vi "Strip HTML.vi"(8 "error in":errorcluster, 11 "HTML String":string) -> (0 "error out":errorcluster, 1 "HTML Stripped String":string, 3 "HTML String OUT":string, 4 "HTML Code Offsets":i32[](array[numeric]), 5 "HTML Codes":string[](array[string]))   [LabVIEW 2017]
doc: "This VI parses an HTML string and removes HTML <...> style tags. The HTML Tag Array contains clusters of the found tags and their corresponding indexes in the original HTML string.\n\nAlso replaces:\n o &nbsp; with \" \" ( a space)\n o &amp; with \"&\"\n\nTypical use of the HTML Tag Array is to locate sections of the HTML code to perform specific operations.\n\nRev 0.0.0 07/09/2009 Phillip Brooks\n Originated."
uses:
  <vilib>/regexp/Match Regular Expression.xnode
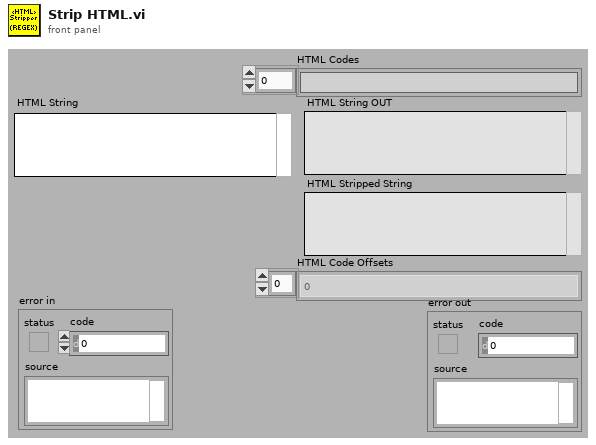
[diagram p1: front panel]
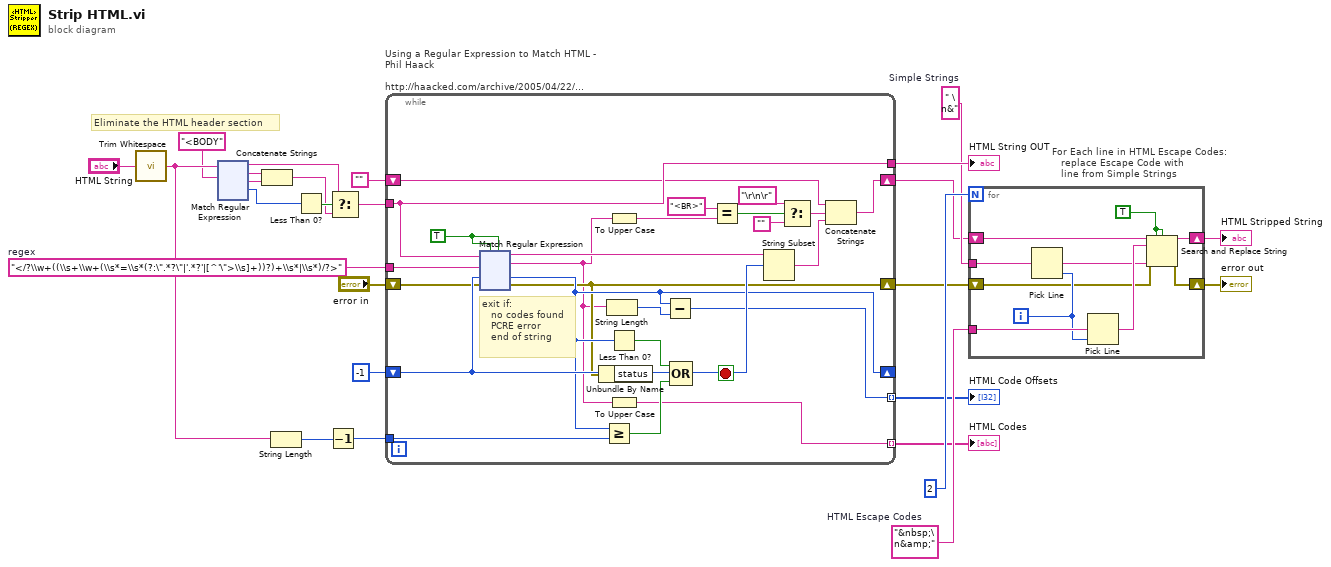
[diagram p0: block diagram]
diagram:
  w17 = " \n&"  # Simple Strings
  w19 = "&nbsp;\n&amp;"  # HTML Escape Codes
  w24 = "</?\\w+((\\s+\\w+(\\s*=\\s*(?:\".*?\"|'.*?'|[^'\">\\s]+))?)+\\s*|\\s*)/?>"  # regex
  # "Eliminate the HTML header section"
  n1 = call <vilib>:"Trim Whitespace.vi"("string"="HTML String") -> ("trimmed string"=w9:string)  [unwired: 1 in]
  n2 = xnode "Match Regular Expression"("input string"=w9, "regular expression"="<BODY") -> ("before match"=w3:string, "whole match"=w6:string, "after match"=w7:string, "offset past match"=w5:i32)  [unwired: 2 in, 3 out]
  n3 = Concatenate Strings(w6, w7) -> (w2:string)
  n4 = String Length(string=w9) -> (length=w22:i32)
  n5 = Less Than 0?(x=w5) -> (x < 0?=w4:bool)
  n6 = Decrement(x=w22) -> (x-1=w21:i32)
  n7 = Select(t=w3, s=w4, f=w2) -> (s? t:f=w1:string)
  n8 = while "Using a Regular Expression to Match HTML - Phil Haack\n\nhttp://haacked.com/archive/2005/04/22/Matching_HTML_With_Regex.aspx" {
    tunnel: w24 -> [w52]
    shift-right: [w44] -> _
    shift-left: -1 -> [w48]
    tunnel: w1 -> [w41]
    shift-right: [w49] -> w16
    shift-left: "" -> [w30]
    tunnel: w21 -> [w43]
    tunnel: [w41] -> w20
    tunnel: [w38] -> w14 mode=indexing
    tunnel: [w39] -> w13 mode=indexing
    shift-right: [w36] -> w11
    shift-left: "error in" -> [w37]
    stop <- w46 stop-if-true
    w40 = TRUE ("ignore case? (F)")
    # "exit if:\n   no codes found\n   PCRE error\n   end of string"
    n9 = xnode "Match Regular Expression"("input string"=w41, "regular expression"=w52, "offset (0)"=w48, "error in"=w37, "ignore case? (F)"=w40, "multiline? (F)"=w40) -> ("before match"=w47:string, "whole match"=w35:string, "offset past match"=w44:i32, "error out"=w36:errorcluster)  [unwired: 1 out]
    n10 = Unbundle By Name(w36) -> ("status"=w45:bool)
    n11 = Greater Or Equal?(x=w44, y=w43) -> (x >= y?=w42:bool)
    n12 = String Length(string=w35) -> (length=w50:i32)
    n13 = To Upper Case(1:w35) -> (0:w33:string)
    n14 = Less Than 0?(x=w44) -> (x < 0?=w51:bool)
    n15 = To Upper Case(1:w35) -> (0:w38:string)
    n16 = Subtract(x=w44, y=w50) -> (x-y=w39:i32)
    n17 = Compound Arithmetic op=OR(w51, w45, w42) -> (w46:bool)
    n18 = Equal?(x="<BR>", y=w33) -> (x = y?=w31:bool)
    n19 = String Subset(string=w47, offset (0)=w48) -> (substring=w34:string)  [unwired: 1 out]
    n20 = Select(t="\r\n\r", s=w31, f="") -> (s? t:f=w28:string)
    n21 = Concatenate Strings(w30, w28, w34) -> (w49:string)
  }
  "HTML String OUT" <- w20
  "HTML Codes" <- w14
  "HTML Code Offsets" <- w13
  n22 = for "For Each line in HTML Escape Codes:\n   replace Escape Code with \n   line from Simple Strings" {
    N: 2 -> [_]
    tunnel: w19 -> [w173]
    shift-right: [w175] -> w15
    shift-left: w16 -> [w174]
    tunnel: w17 -> [w170]
    shift-right: [w167] -> w10
    shift-left: w11 -> [w168]
    i -> [w169]
    w176 = TRUE ("replace all? (F)")
    n23 = Pick Line(multi-line string=w170, line index=w169) -> (output string=w171:string)  [unwired: 1 out]
    n24 = Pick Line(multi-line string=w173, line index=w169) -> (output string=w172:string)  [unwired: 1 out]
    n25 = Search and Replace String(replace all?=w176, case sensitive?=w176, input string=w174, search string=w172, replace string=w171, error in=w168) -> (result string=w175:string, error out=w167:errorcluster)  [unwired: 1 in, 3 out]
  }
  "HTML Stripped String" <- w15
  "error out" <- w10
